vi "XML Script - Control.vi"   [LabVIEW 2020]
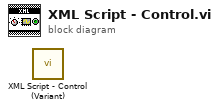
[diagram p0: block diagram]
diagram:
  n1 = call <vilib>:"XML Script - Control (Variant).vi"() -> ()  [unwired: 10 in, 2 out]
